vi "mxwScript_API_SetVal_LoneExternalNodeState.vi"(8 "error in (no error)":errorcluster, 11 "external node state":variant) -> (0 "error out":errorcluster, 3 "parameter":T1)   [LabVIEW 2020]
uses:
  codeGenAPISupport.llb/cgAPI_mxwScript_Parameter.ctl
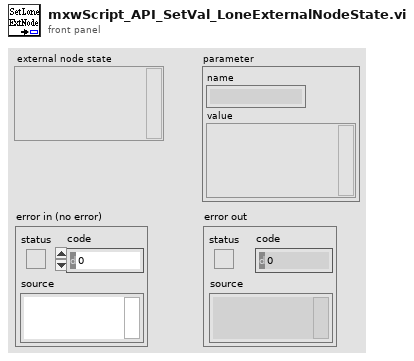
[diagram p1: front panel]
types:
  T1 = typedef "cgAPI_mxwScript_Parameter.ctl" = cluster{"name":string, "value":variant}
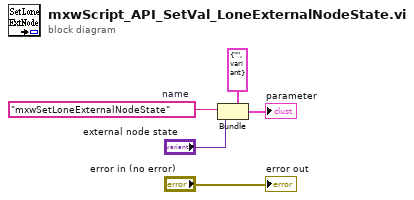
[diagram p0: block diagram]
diagram:
  w2 = "mxwSetLoneExternalNodeState"  # name
  n1 = Bundle(cluster=T1 {"name"="", "value"=variant} ("parameter"), "name"=w2, "value"="external node state") -> (→"parameter":T1)
  "error out" <- "error in (no error)"
